vi "Configure Controller Normal Response.vi"(8 "error in (no error)":errorcluster, 9 "normal response":u8=128, 10 "node":u8, 11 "ProPar in":refnum<class "PL Bronkhorst ProPar.lvclass">) -> (0 "error out":errorcluster, 3 "ProPar out":refnum<class "PL Bronkhorst ProPar.lvclass">)   [LabVIEW 2015, in "PL Bronkhorst ProPar.lvclass"]
doc: "Configures controller response during normal control of the specified <b>node</b>. Value 128 means no correction."
uses:
  PL Bronkhorst ProPar.lvclass
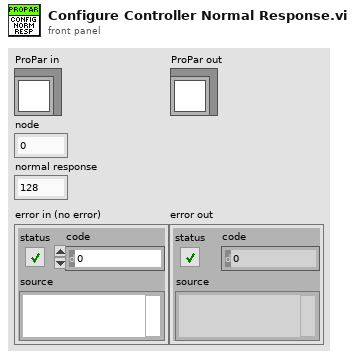
[diagram p1: front panel]
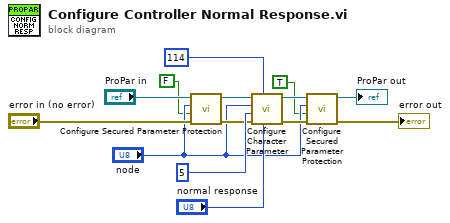
[diagram p0: block diagram]
diagram:
  n1 = call "Configure Secured Parameter Protection.vi"("error in (no error)"="error in (no error)", "enable protection"=FALSE, "node"="node", "ProPar in"="ProPar in") -> ("error out"=w5:errorcluster, "ProPar out"=w6:refnum<class "PL Bronkhorst ProPar.lvclass">)  [unwired: 6 in]
  n2 = call "Configure Character Parameter.vi"("value"="normal response", "process number"=u8 114, "error in (no error)"=w5, "parameter number"=u8 5 ("process number"), "node"="node", "ProPar in"=w6) -> ("error out"=w9:errorcluster, "ProPar out"=w10:refnum<class "PL Bronkhorst ProPar.lvclass">)  [unwired: 4 in]
  n3 = call "Configure Secured Parameter Protection.vi"("error in (no error)"=w9, "enable protection"=TRUE, "node"="node", "ProPar in"=w10) -> ("error out"=→"error out":errorcluster, "ProPar out"=→"ProPar out":refnum<class "PL Bronkhorst ProPar.lvclass">)  [unwired: 6 in]
